vi "e.gate TimeFormatHeader.vi"(10 "String":string) -> (2 "Date/Time HeaderArray":string[](array[string]))   [LabVIEW 2009]
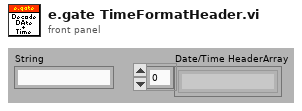
[diagram p1: front panel]
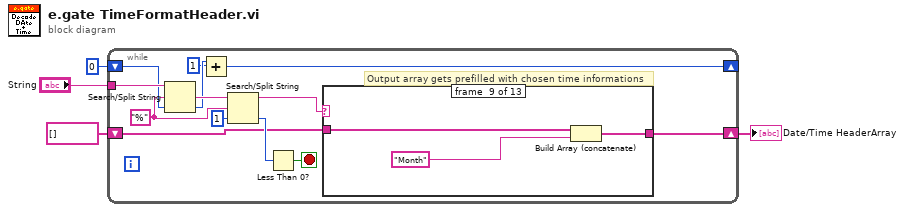
[diagram p0: block diagram]
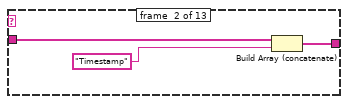
[diagram p3: hidden frame]
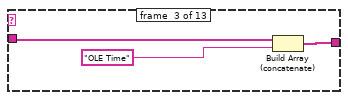
[diagram p4: hidden frame]
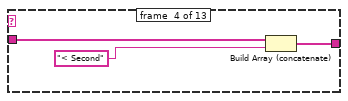
[diagram p5: hidden frame]
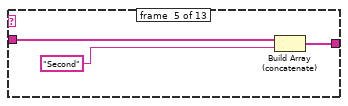
[diagram p6: hidden frame]
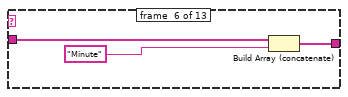
[diagram p7: hidden frame]
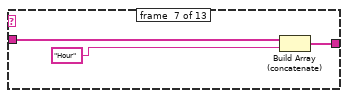
[diagram p8: hidden frame]
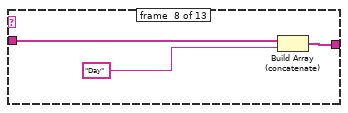
[diagram p9: hidden frame]
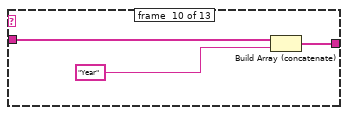
[diagram p10: hidden frame]
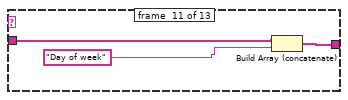
[diagram p11: hidden frame]
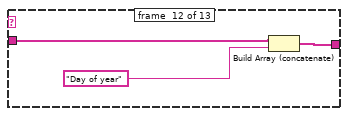
[diagram p12: hidden frame]
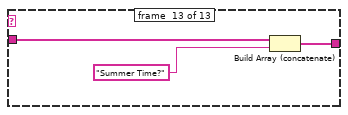
[diagram p13: hidden frame]
diagram:
  n1 = while {
    shift-right: [w17] -> w2
    shift-left: string[] [] -> [w5]
    tunnel: "String" -> [w16]
    shift-right: [w8] -> _
    shift-left: 0 -> [w15]
    stop <- w10 stop-if-true
    w12 = "%" ("Nach String/Zeichen suchen (-)")
    # "Output array gets prefilled with chosen time informations"
    n2 = Search/Split String(string=w16, search string/char (-)=w12, offset (0)=w15) -> (match + rest of string=w14:string, offset of match=w7:i32)  [unwired: 1 out]
    n3 = Add ("Addieren")(x=w7, y=1) -> (x+y=w8:i32)
    n4 = Search/Split String(string=w14, search string/char (-)=w12, offset (0)=1 ("Offset (0)")) -> (substring before match=w11:string, offset of match=w9:i32)  [unwired: 1 out]
    n5 = Less Than 0?(x=w9) -> (x < 0?=w10:bool)
    n6 = case shown="\"%ST\"" w11 {
      tunnel: w5 -> [w18 w20 w24 w27 w30 w33 w36 w39 w42 w45 w48 w51 w54]
      tunnel: [w18 w21 w23 w26 w29 w32 w35 w38 w41 w44 w47 w50 w53] -> w17
      frame #0 {
      }
      frame #1 {
        n7 = Build Array (concatenate)(w20, "Timestamp" ("Nach String/Zeichen suchen (-)")) -> (w21:string[])
      }
      frame #2 {
        n8 = Build Array (concatenate)(w24, "OLE Time" ("Nach String/Zeichen suchen (-)")) -> (w23:string[])
      }
      frame #3 {
        n9 = Build Array (concatenate)(w27, "< Second" ("Nach String/Zeichen suchen (-)")) -> (w26:string[])
      }
      frame #4 {
        n10 = Build Array (concatenate)(w30, "Second" ("Nach String/Zeichen suchen (-)")) -> (w29:string[])
      }
      frame #5 {
        n11 = Build Array (concatenate)(w33, "Minute" ("Nach String/Zeichen suchen (-)")) -> (w32:string[])
      }
      frame #6 {
        n12 = Build Array (concatenate)(w36, "Hour" ("Nach String/Zeichen suchen (-)")) -> (w35:string[])
      }
      frame #7 {
        n13 = Build Array (concatenate)(w39, "Day" ("Nach String/Zeichen suchen (-)")) -> (w38:string[])
      }
      frame #8 {
        n14 = Build Array (concatenate)(w42, "Month" ("Nach String/Zeichen suchen (-)")) -> (w41:string[])
      }
      frame #9 {
        n15 = Build Array (concatenate)(w45, "Year" ("Nach String/Zeichen suchen (-)")) -> (w44:string[])
      }
      frame #10 {
        n16 = Build Array (concatenate)(w48, "Day of week" ("Nach String/Zeichen suchen (-)")) -> (w47:string[])
      }
      frame #11 {
        n17 = Build Array (concatenate)(w51, "Day of year" ("Nach String/Zeichen suchen (-)")) -> (w50:string[])
      }
      frame #12 {
        n18 = Build Array (concatenate)(w54, "Summer Time?" ("Nach String/Zeichen suchen (-)")) -> (w53:string[])
      }
    }
  }
  "Date/Time HeaderArray" <- w2
